vi "ViewCapture.vi"(8 "error in (no error)":errorcluster, 10 "Open":bool, 11 "DCIMG Path":path) -> (0 "error out":errorcluster)   [LabVIEW 2012]
panel:
  out "Image":u16[][](graph)
  out "Time Stamp":dbl
  in  "Index":i32 min=0 max=99 step=1
  out "Total":i32
  in  "Quit":bool
  out "Openfile":bool
  in  "Frame Index":i32(c297)
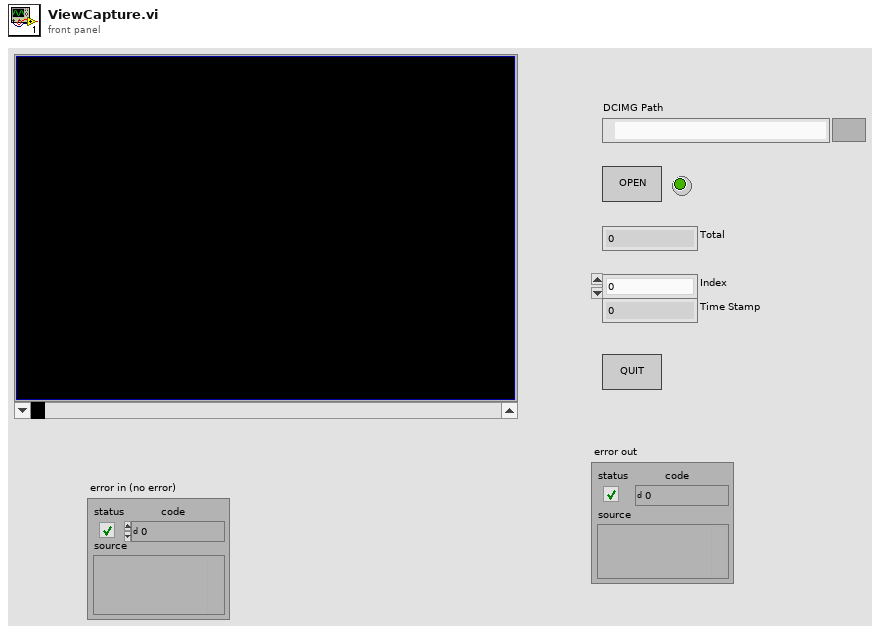
[diagram p1: front panel]
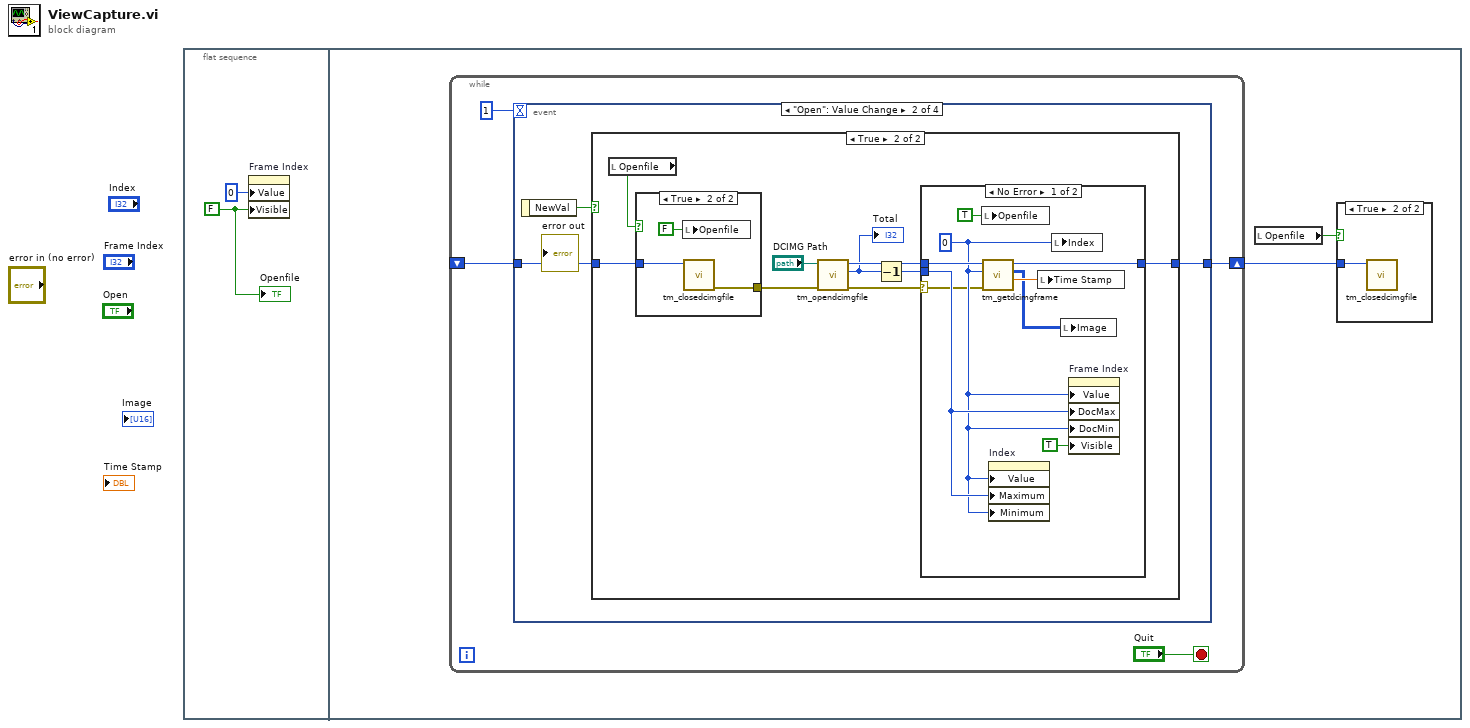
[diagram p0: block diagram]
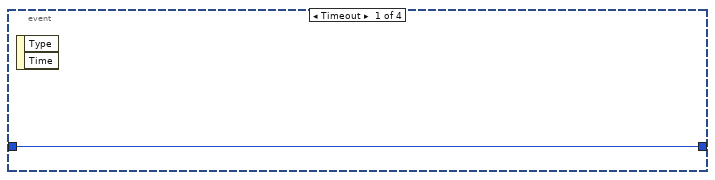
[diagram p3: hidden frame]
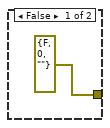
[diagram p5: hidden frame]
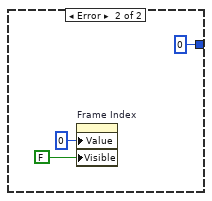
[diagram p6: hidden frame]
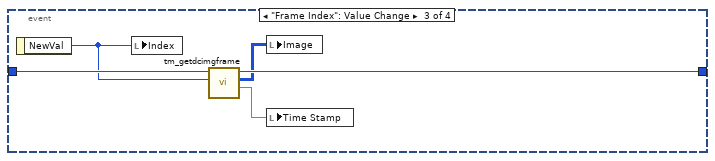
[diagram p7: hidden frame]
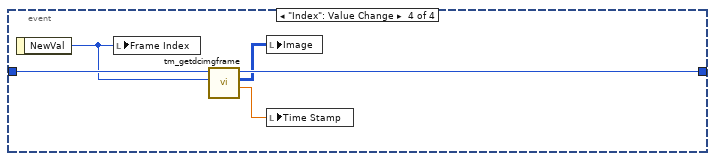
[diagram p8: hidden frame]
diagram:
  n1 = flat-sequence {
    frame #0 {
      w1 = FALSE ("Visible")
      n2 = property on="Frame Index" class="Scroll (strict)"("Value"=0 ("Frame Index"), "Visible"=w1) -> ()  [unwired: 2 in, 2 out]
      "Openfile" <- w1
    }
    frame #1 {
      n3 = while {
        shift-right: [w9] -> w3
        shift-left: _ -> [w8]
        stop <- "Quit" stop-if-true
        n4 = event shown="[1] \"Open\": Value Change" {
          selector: _ -> [_ _ _ _]
          dyn-events: _ -> [_ _ _ _]
          timeout: 1 -> [_ _ _ _]
          tunnel: [w10 w12 w43 w48] -> w9
          tunnel: w8 -> [w10 w11 w44 w49]
          event Timeout {
            n5 = event-data() -> ()  [unwired: 1 in, 2 out]
          }
          event "Open": Value Change {
            n6 = event-data() -> ("NewVal"=w13:bool)  [unwired: 1 in]
            n7 = case shown="True" w13 {
              tunnel: [w14 w21] -> w12
              tunnel: w11 -> [w14 w20]
              frame False {
              }
              frame True {
                n8 = local read "Openfile"() -> (w19:bool)
                n9 = case shown="True" w19 {
                  tunnel: w20 -> [_ w27]
                  tunnel: [errorcluster {"status"=FALSE, "code"=0, "source"=""} ("error out") w25] -> w18
                  frame False {
                  }
                  frame True {
                    n10 = local write "Openfile"(FALSE ("Openfile")) -> ()
                    n11 = call <userlib>:"tm_closedcimgfile.vi"("File Handle"=w27) -> ("error out"=w25:errorcluster)  [unwired: 10 in]
                  }
                }
                n12 = call <userlib>:"tm_opendcimgfile.vi"("error in (no error)"=w18, "Path"="DCIMG Path") -> ("error out"=w17:errorcluster, "Total Frames"=w16:i32, "File Handle"=w22:u32)  [unwired: 7 in]
                "Total" <- w16
                n13 = Decrement(x=w16) -> (x-1=w15:i32)
                n14 = case shown="No Error" w17 {
                  selector: w17 -> [w29 _]
                  tunnel: w22 -> [w36 _]
                  tunnel: w15 -> [w31 _]
                  tunnel: [w35 u32 0 ("File Handle out")] -> w21
                  frame No Error {
                    w30 = 0 ("Frame Index")
                    n15 = local write "Openfile"(TRUE ("Openfile")) -> ()
                    n16 = call <userlib>:"tm_getdcimgframe.vi"("error in (no error)"=w29, "Frame Index"=w30, "File Handle in"=w36) -> ("Time Sec"=w32:dbl, "Data"=w28:u16[][], "File Handle out"=w35:u32)  [unwired: 5 in, 1 out]
                    n17 = property on="Index" class="DigNum (strict)"("Value"=w30, "Maximum"=w31, "Minimum"=w30) -> ()  [unwired: 2 in, 2 out]
                    n18 = local write "Time Stamp"(w32) -> ()
                    n19 = local write "Index"(w30) -> ()
                    n20 = local write "Image"(w28) -> ()
                    n21 = property on="Frame Index" class="Scroll (strict)"("Value"=w30, "DocMax"=w31, "DocMin"=w30, "Visible"=TRUE) -> ()  [unwired: 2 in, 2 out]
                  }
                  frame Error {
                    n22 = property on="Frame Index" class="Scroll (strict)"("Value"=0 ("Frame Index"), "Visible"=FALSE) -> ()  [unwired: 2 in, 2 out]
                  }
                }
              }
            }
          }
          event "Frame Index": Value Change {
            n23 = event-data() -> ("NewVal"=w42:i32)  [unwired: 1 in]
            n24 = local write "Index"(w42) -> ()
            n25 = call <userlib>:"tm_getdcimgframe.vi"("Frame Index"=w42, "File Handle in"=w44) -> ("Time Sec"=w40:dbl, "Data"=w41:u16[][], "File Handle out"=w43:u32)  [unwired: 6 in, 1 out]
            n26 = local write "Image"(w41) -> ()
            n27 = local write "Time Stamp"(w40) -> ()
          }
          event "Index": Value Change {
            n28 = event-data() -> ("NewVal"=w47:i32)  [unwired: 1 in]
            n29 = local write "Frame Index"(w47) -> ()
            n30 = call <userlib>:"tm_getdcimgframe.vi"("Frame Index"=w47, "File Handle in"=w49) -> ("Time Sec"=w45:dbl, "Data"=w46:u16[][], "File Handle out"=w48:u32)  [unwired: 6 in, 1 out]
            n31 = local write "Image"(w46) -> ()
            n32 = local write "Time Stamp"(w45) -> ()
          }
        }
      }
      n33 = local read "Openfile"() -> (w4:bool)
      n34 = case shown="True" w4 {
        tunnel: w3 -> [_ w5]
        frame False {
        }
        frame True {
          n35 = call <userlib>:"tm_closedcimgfile.vi"("File Handle"=w5) -> ()  [unwired: 10 in, 1 out]
        }
      }
    }
  }
